vi "Check if Executable program.vi"(1 "error in (no error)":errorcluster) -> (0 "error out":errorcluster)   [LabVIEW 2018]
doc: "Revision: 11.05.97\nDescription: Exit program if it is an executable\nGlobals: None\nWrite:None\nOccurrences: none\nDevices: none\nFiles: none\nSystem: none"
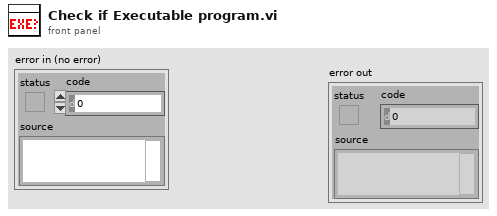
[diagram p1: front panel]
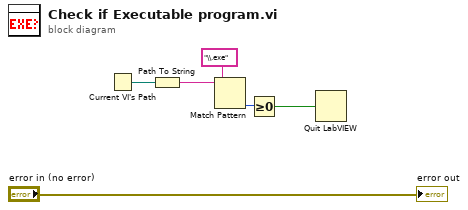
[diagram p0: block diagram]
diagram:
  n1 = Current VI's Path() -> (path=w3:path)
  n2 = Path To String(path=w3) -> (string=w2:string)
  n3 = Match Pattern(string=w2, regular expression="\\.exe") -> (offset past match=w5:i32)  [unwired: 1 in, 3 out]
  n4 = Greater Or Equal To 0?(x=w5) -> (x >= 0?=w1:bool)
  n5 = Quit LabVIEW(quit? (T)=w1) -> ()
  "error out" <- "error in (no error)"
